vi "Lift Control. Inc.vi"() -> ()   [LabVIEW 2014]
uses:
  Text Variable VIs/Read Number Variable.vi
  <vilib>/Rock Robotics/WPI/MotorControl/WPI_MotorControlOpen Talon.vi
  SRE Enum.ctl
panel:
  out "Bot Switch On":bool
  in  "Motor":dbl
  in  "Enum":T1
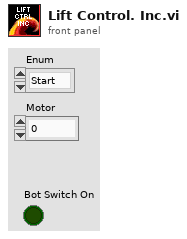
[diagram p1: front panel]
types:
  T1 = typedef "SRE Enum.ctl" = enum16{"Start", "Run", "End"}
  T2 = typedef "WPI_MotorControlDeviceRef.ctl" = cluster{"DeviceStatus":errorcluster, "Type":T3, "PWM":cluster{"Controller":T4, "PWM Channel":T5, "DeadBand":T6}, "CAN":cluster{"Device Number":u8, "Control Mode":T7, "Semaphore":T8, "Max Vout":dbl, "TalonSRX Control Mode":T9}, "Invert":bool, "TransformRef":T10, "InvTransformRef":T10}
  T3 = typedef "WPI_MotorControlType.ctl" = enum16{"PWM", "CAN", "CANTalonSRX"}
  T4 = typedef "FPGA_TypedefDigitalModule.ctl" = enum16{"Controller 1"}
  T5 = typedef "FPGA_DIOPWMChannel.ctl" = enum8{"PWM 0", "PWM 1", "PWM 2", "PWM 3", "PWM 4", "PWM 5", "PWM 6", "PWM 7", "PWM 8", "PWM 9", "PWM MXP 0", "PWM MXP 1", "PWM MXP 2", "PWM MXP 3", "PWM MXP 4", "PWM MXP 5", "PWM MXP 6", "PWM MXP 7", "PWM MXP 8", "PWM MXP 9", "Invalid"}
  T6 = typedef "WPI_PWMDeadband.ctl" = cluster{"Name":string, "maxPositivePwm":i32, "minPositivePwm":i32, "centerPwm":i32, "maxNegativePwm":i32, "minNegativePwm":i32, "angularRange":u16}
  T7 = typedef "WPI_CANJaguar_ControlMode.ctl" = enum8{"Percent VBus", "Current", "Speed", "Position", "Voltage"}
  T8 = typedef "Semaphore RefNum" = refnum<k1>
  T9 = typedef "WPI_CANTalonSRX_APIControlMode.ctl" = enum8{"Percent VBus", "Speed", "Position", "Slave", "Unchanged / Invalid"}
  T10 = typedef "WPI_PWMTransform_ConPane.ctl" = refnum<vi>
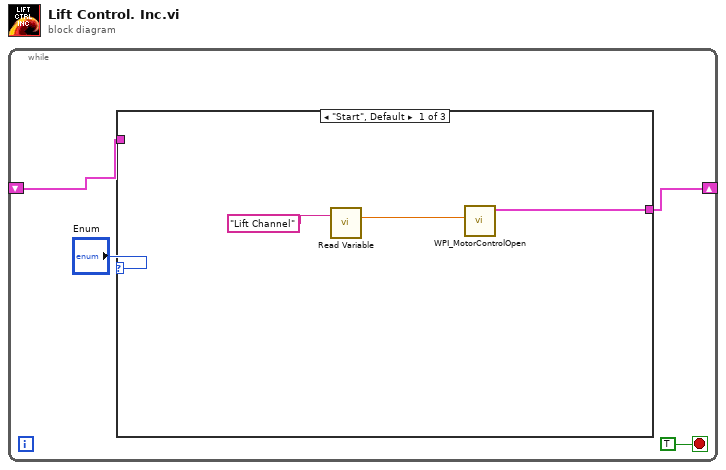
[diagram p0: block diagram]
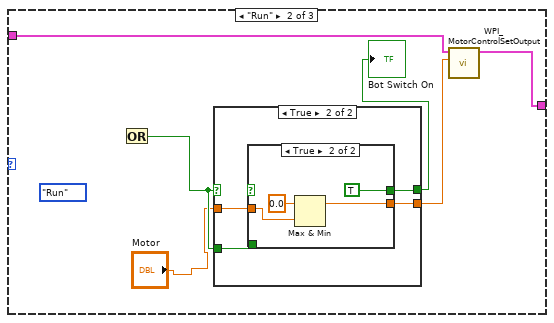
[diagram p2: hidden frame]
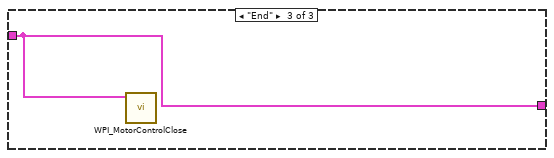
[diagram p5: hidden frame]
diagram:
  n1 = while {
    shift-right: [w3] -> _
    shift-left: _ -> [w2]
    stop <- TRUE stop-if-true
    n2 = case shown="\"Start\", Default" "Enum" {
      tunnel: [w5 w9 w22] -> w3
      tunnel: w2 -> [_ w8 w22]
      frame "Start", Default {
        n3 = call-poly "Read Variable.vi"("Name"="Lift Channel") -> ("number"=w6:dbl)  [unwired: 1 in, 1 out]
        n4 = call-poly <vilib>:"WPI_MotorControlOpen.vi"("PWM Channel"=w6) -> ("MotorControlDeviceRef"=w5:T2)  [unwired: 9 in, 1 out]
      }
      frame "Run" {
        (unwired) SRE_Enum."Run" ("Enum")
        n5 = Or() -> (x .or. y?=w13:bool)  [unwired: 2 in]
        n6 = case shown="True" w13 {
          tunnel: [_ w17] -> w10
          tunnel: w13 -> [_ w16]
          tunnel: "Motor" -> [_ w15]
          tunnel: [_ w14] -> w11
          frame False {
          }
          frame True {
            n7 = case shown="True" {
              selector: _ -> [_ _]
              tunnel: [_ TRUE] -> w17
              tunnel: w16 -> [_ _]
              tunnel: w15 -> [_ w20]
              tunnel: [_ w18] -> w14
              frame False {
              }
              frame True {
                n8 = Max & Min(x=0.0, y=w20) -> (max(x,y)=w18:dbl)  [unwired: 1 out]
              }
            }
          }
        }
        "Bot Switch On" <- w10
        n9 = call <vilib>:"WPI_MotorControlSetOutput.vi"("Output"=w11, "MotorControlDevRef"=w8) -> ("MotorControlDevRef"=w9:T2)  [unwired: 7 in, 2 out]
      }
      frame "End" {
        n10 = call <vilib>:"WPI_MotorControlClose.vi"("MotorControlDevRef"=w22) -> ()  [unwired: 10 in, 1 out]
      }
    }
  }
